vi "SolveIKPosition.vi"(4 "error in":errorcluster, 5 "Pose":T2={"Position"={"x"=0.457, "y"=-0.385, "z"=-0.261}, "Orientation"={"Roll (y)"=3.13, "Pitch (x)"=-0.1, "Yaw (z)"=-1.85}}, 6 "Side":T3, 7 "node":string) -> (0 "error out":errorcluster)   [LabVIEW 2010]
uses:
  ROS/MessageBuilding/std_msgs/subs/u32Scalar.vi
  ROS/Code/SubVIs/_ROSDirection.ctl
  ROS/Code/Console/Servers/ServerSubs/TopicDef.ctl
  ROS/Code/SubVIs/BaxterSide.ctl
panel:
  out "IK Reply":T1
  out "Reply":string
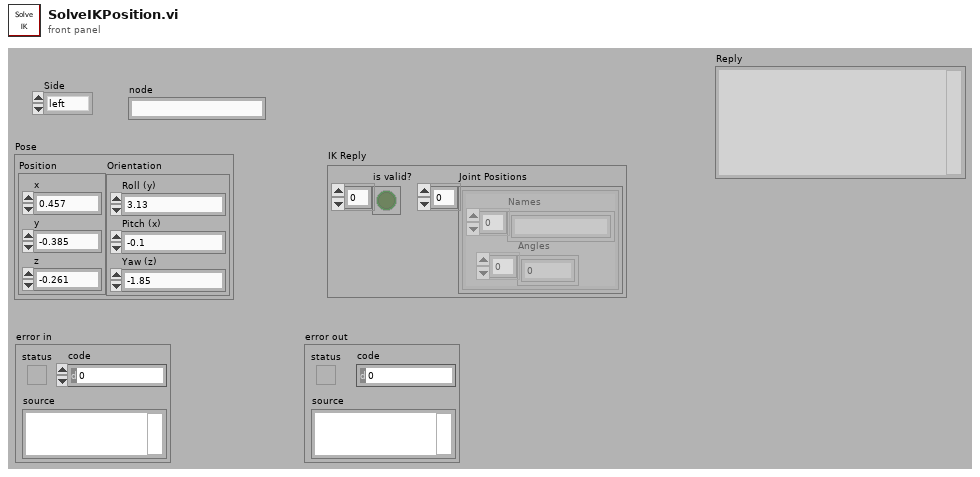
[diagram p1: front panel]
types:
  T1 = cluster{"is valid?":bool[], "Joint Positions":cluster{"Angles":dbl[], "Names":string[]}[]}
  T2 = cluster{"Position":cluster{"x":dbl, "y":dbl, "z":dbl}, "Orientation":cluster{"Roll (y)":dbl, "Pitch (x)":dbl, "Yaw (z)":dbl}}
  T3 = typedef "BaxterSide.ctl" = enum16{"left", "right"}
  T4 = typedef "TopicDef.ctl" = cluster{"Topic":string, "Type":string, "Action":T5, "Update (ms)":u16, "write queue":u16}
  T5 = typedef "_ROSDirection.ctl" = enum16{"Node", "Publisher", "Subscriber", "Service Client"}
  T6 = cluster{"Roll (y)":dbl, "Pitch (x)":dbl, "Yaw (z)":dbl}
  T7 = typedef "_ROSControl.ctl" = cluster{"topic port":u16, "Node":string, "topic":string, "type":string, "node port":u32, "error ":errorcluster, "Direction":T5, "APIs":string[], "Update (ms)":u16, "write queue":u16}
  T8 = cluster{"Position":cluster{"x":dbl, "y":dbl, "z":dbl}, "Quaternion":cluster{"x":dbl, "y":dbl, "z":dbl, "w":dbl}}
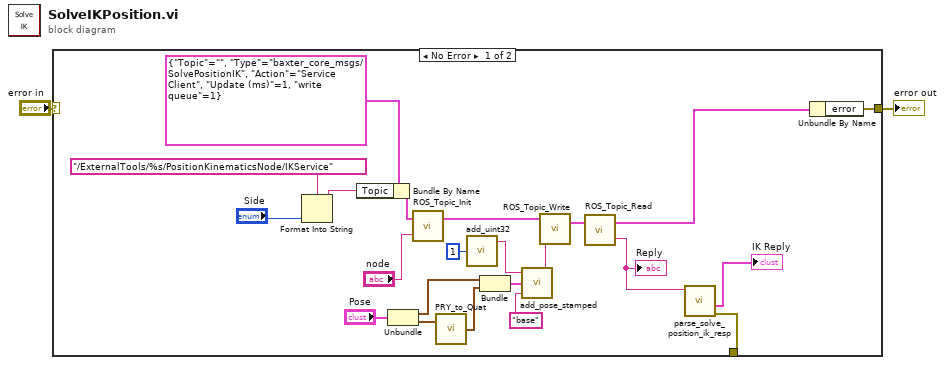
[diagram p0: block diagram]
diagram:
  n1 = case shown="No Error" "error in" {
    selector: "error in" -> [_ w25]
    tunnel: [w24 w25] -> w2
    tunnel: [w10 _] -> _
    frame No Error {
      n2 = Format Into String(format string="/ExternalTools/%s/PositionKinematicsNode/IKService" ("topic"), "Side") -> (resulting string=w7:string)  [unwired: 2 in, 1 out]
      n3 = Bundle By Name(cluster=T4 {"Topic"="", "Type"="baxter_core_msgs/SolvePositionIK", "Action"=enum."Service Client", "Update (ms)"=1, "write queue"=1} ("Definitions"), "Topic"=w7) -> (w3:T4)
      n4 = Unbundle("Pose") -> ("Position"=w18:cluster{"x":dbl, "y":dbl, "z":dbl}, "Orientation"=w20:T6)
      n5 = call "ROS_Topic_Init.vi"("node"="node", "Definitions"=w3) -> ("ROS out"=w12:T7)  [unwired: 1 in]
      n6 = call "PRY_to_Quat.vi"("Orientation"=w20) -> ("Quaternion"=w19:cluster{"x":dbl, "y":dbl, "z":dbl, "w":dbl})  [unwired: 1 in]
      n7 = call-poly "add_uint32.vi"("Numeric"=u32 1) -> ("msg out"=w13:string)  [unwired: 4 in]
      n8 = Bundle("Position"=w18, "Quaternion"=w19) -> (w17:T8)  [unwired: 1 in]
      n9 = call "add_pose_stamped.vi"("frame_id"="base", "Pose"=w17, "msg in"=w13) -> ("msg out"=w14:string)  [unwired: 2 in]
      n10 = call "ROS_Topic_Write.vi"("Msg in"=w14, "ROS in"=w12) -> ("ROS out"=w8:T7)  [unwired: 2 in]
      n11 = call "ROS_Topic_Read.vi"("ROS in"=w8) -> ("Reply"=w11:string, "ROS out"=w22:T7)  [unwired: 1 in]
      "Reply" <- w11
      n12 = call "parse_solve_position_ik_resp.vi"("msg in"=w11) -> ("error out"=w10:errorcluster, "IK Reply"=→"IK Reply":T1)  [unwired: 3 in, 2 out]
      n13 = Unbundle By Name(w22) -> ("error"=w24:errorcluster)
    }
    frame Error {
    }
  }
  "error out" <- w2
